vi "Read Properties.vi"(8 "error in":errorcluster, 11 "Report Viewer in":refnum<class "Report Viewer.lvclass">) -> (0 "error out":errorcluster, 3 "Report Viewer out":refnum<class "Report Viewer.lvclass">)   [LabVIEW 2023, in "Report Viewer.lvlib" / "Report Viewer.lvclass"]
uses:
  Library/Report Viewer.lvclass
  Library/Report Viewer.lvclass/Report Viewer.ctl
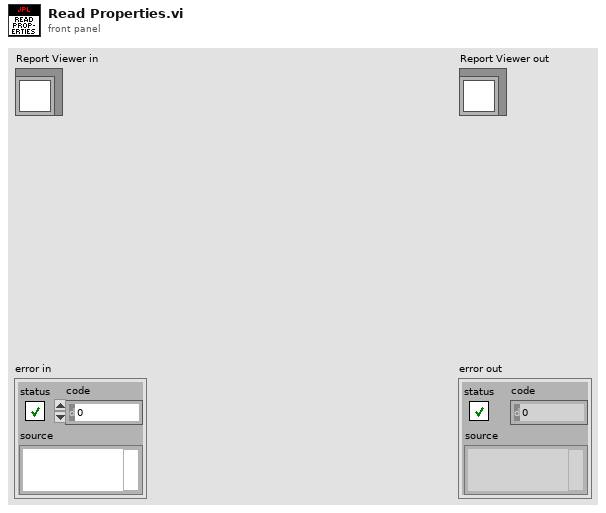
[diagram p1: front panel]
types:
  T1 = typedef "Report Viewer.lvlib/Report Viewer.lvclass/Data to Read.ctl" = cluster{"Group":string, "Channel":string}
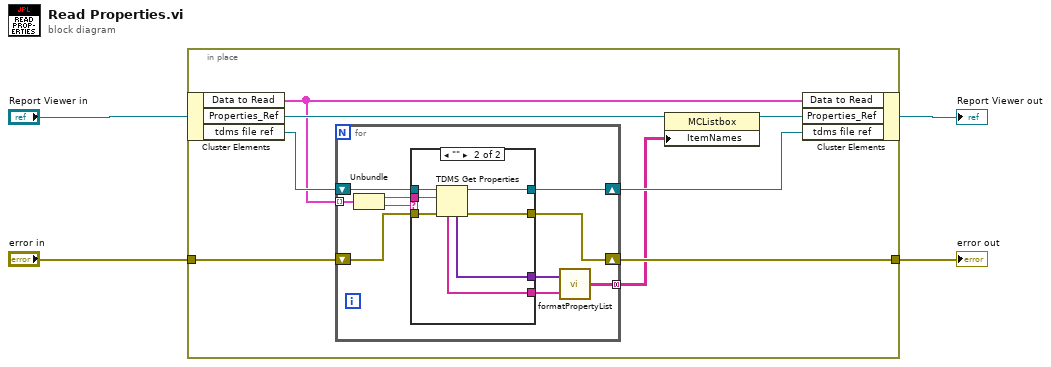
[diagram p0: block diagram]
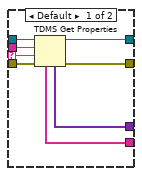
[diagram p2: hidden frame]
diagram:
  n1 = in-place {
    in-place-border: "error in" -> [w10]
    in-place-border: [w9] -> w1
    n2 = in-place-cluster #1("Report Viewer in") -> ("Data to Read"=w5:T1[], "Properties_Ref"=w8:refnum<vi>, "tdms file ref"=w12:refnum<k34>)
    n3 = for {
      shift-right: [w21] -> w11
      shift-left: w12 -> [w22]
      tunnel: w5 -> [w20] mode=indexing
      shift-right: [w17] -> w9
      shift-left: w10 -> [w18]
      tunnel: [w16] -> w6 mode=concatenating
      n4 = Unbundle(w20) -> ("Group"=w19:string, "Channel"=w13:string)
      n5 = case shown="\"\"" w13 {
        selector: w13 -> [w23 _]
        tunnel: w22 -> [w30 w37]
        tunnel: [w29 w36] -> w21
        tunnel: w19 -> [w28 w35]
        tunnel: w18 -> [w27 w34]
        tunnel: [w26 w33] -> w17
        tunnel: [w25 w32] -> w15
        tunnel: [w24 w31] -> w14
        frame Default {
          n6 = TDMS Get Properties(8:w27, 9:w23, 10:w28, 11:w30) -> (0:w26:errorcluster, 3:w29:refnum<k34>, 4:w25:variant[], 6:w24:string[])  [unwired: 2 in, 2 out]
        }
        frame "" {
          n7 = TDMS Get Properties(8:w34, 10:w35, 11:w37) -> (0:w33:errorcluster, 3:w36:refnum<k34>, 4:w32:variant[], 6:w31:string[])  [unwired: 3 in, 2 out]
        }
      }
      n8 = call <vilib>:"formatPropertyList.vi"("property names"=w14, "property values"=w15) -> ("strings"=w16:string[][])
    }
    n9 = property class="MCListbox"(reference=w8, "ItemNames"=w6) -> (reference out=w7:refnum<vi>)  [unwired: 1 in, 1 out]
    n10 = in-place-cluster #1("Data to Read"=w5, "Properties_Ref"=w7, "tdms file ref"=w11) -> (→"Report Viewer out":refnum<class "Report Viewer.lvclass">)
  }
  "error out" <- w1
